vi "GetDeviceByType.vi"(8 "error in (no error)":errorcluster, 11 "DevType":i32) -> (0 "error out":errorcluster, 2 "UniqueIDs":string[](array[string]), 3 "Names":string[](array[string]))   [LabVIEW 2009]
doc: "JYGetMonos.vi\nInput - Input Error Cluster\n----------------------------------\n\nOutputs -\nUniquedIDs - string array\nDisplayNames - string array\nOutput Error Cluster\n\nUses the JYConfiguration Browser return a list\nof registered monos.\n\nThe UniqueID will be required to initialize\nthe mono"
panel:
  in  "Config Browser":refnum<k7>
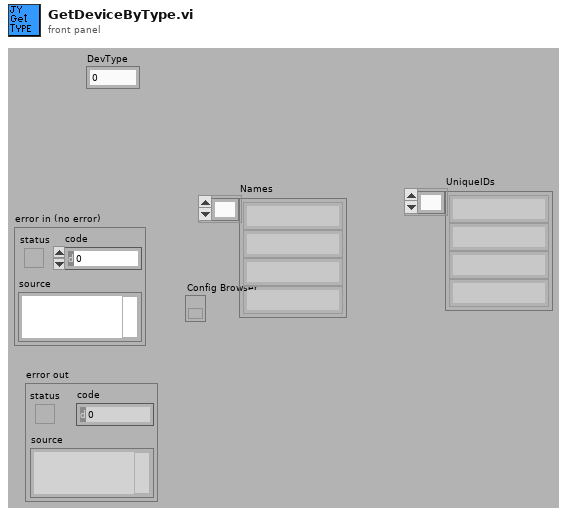
[diagram p1: front panel]
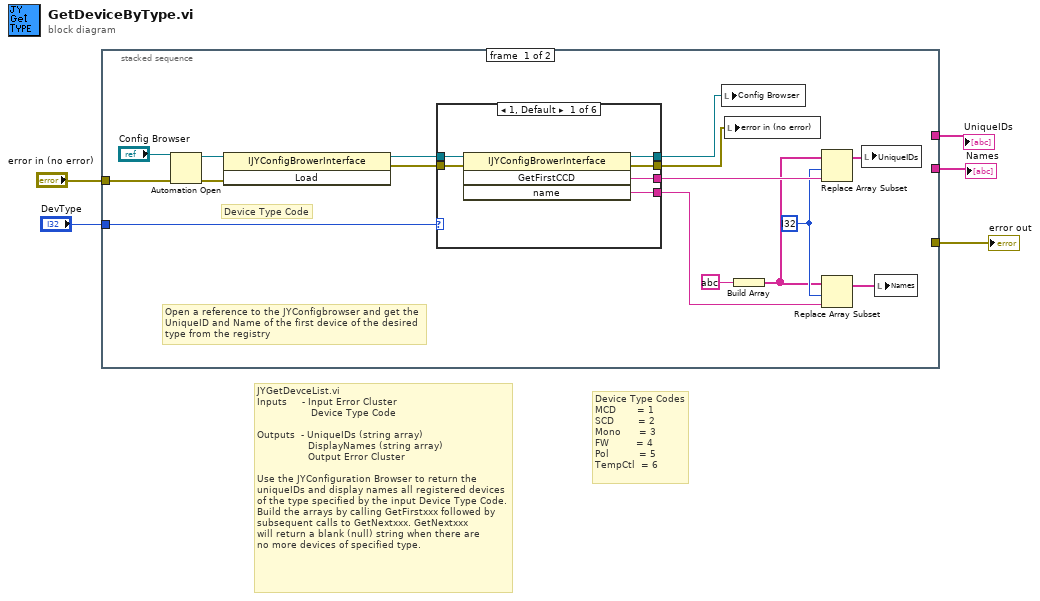
[diagram p0: block diagram]
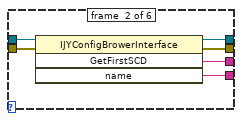
[diagram p2: hidden frame]
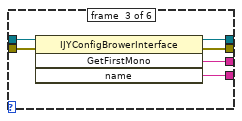
[diagram p3: hidden frame]
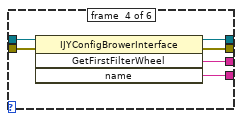
[diagram p4: hidden frame]
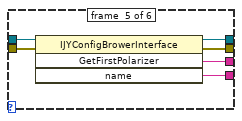
[diagram p5: hidden frame]
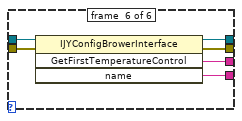
[diagram p6: hidden frame]
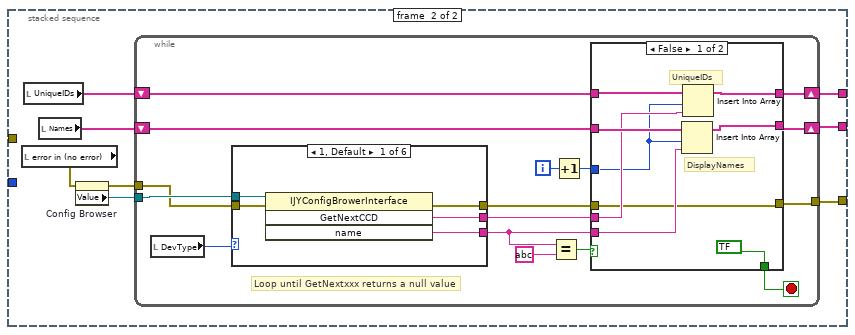
[diagram p7: hidden frame]
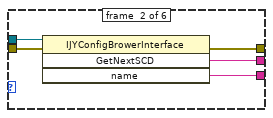
[diagram p8: hidden frame]
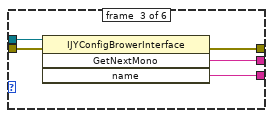
[diagram p9: hidden frame]
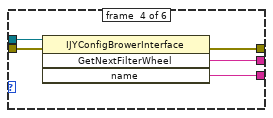
[diagram p10: hidden frame]
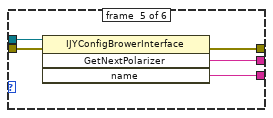
[diagram p11: hidden frame]
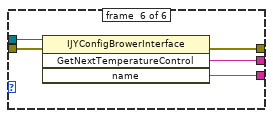
[diagram p12: hidden frame]
diagram:
  # "Device Type Codes\nMCD       = 1\nSCD        = 2\nMono      = 3\nFW         = 4\nPol          = 5\nTempCtl  = 6"
  # "JYGetDevceList.vi\nInputs     - Input Error Cluster\n                  Device Type Code\n\nOutputs  - UniqueIDs (string array)\n                 DisplayNames (string array)\n                 Output Error Cluster\n\nUse the JYConfiguration Browser to return the\nuniqueIDs and display names all registered devices\nof the type specified by the input Device Type Code.\nBuild the arrays by calling GetFirstxxx followed by\nsubsequent calls to GetNextxxx. GetNextxxx\nwill return a blank (null) string when there are\nno more devices of specified type."
  n1 = stacked-sequence {
    tunnel: [_ w60] -> w4
    tunnel: [_ w59] -> w5
    tunnel: [_ w58] -> w2
    tunnel: "error in (no error)" -> [w7 _]
    tunnel: "DevType" -> [w6 _]
    frame #0 {
      w12 = i32 ?
      # "Device Type Code"
      # "Open a reference to the JYConfigbrowser and get the\nUniqueID and Name of the first device of the desired\ntype from the registry"
      n2 = Automation Open(error in (no error)=w7, Automation Refnum="Config Browser") -> (Automation Refnum=w21:refnum<k7>, error out=w19:errorcluster)  [unwired: 2 out]
      n3 = invoke class="IJYConfigBrowerInterface" method="Load"(reference=w21, error in=w19) -> (reference out=w20:refnum<k7>, error out=w18:errorcluster)  [unwired: 1 in, 1 out]
      n4 = case shown="1, Default" w6 {
        tunnel: w20 -> [w22 w33 w39 w45 w51 w57]
        tunnel: w18 -> [w27 w32 w38 w44 w50 w56]
        tunnel: [w26 w31 w37 w43 w49 w55] -> w16
        tunnel: [w25 w30 w36 w42 w48 w54] -> w14
        tunnel: [w24 w29 w35 w41 w47 w53] -> w13
        tunnel: [w23 w28 w34 w40 w46 w52] -> w10
        frame #0 {
          n5 = invoke class="IJYConfigBrowerInterface" method="GetFirstCCD"(reference=w22, error in=w27) -> (reference out=w26:refnum<k7>, error out=w25:errorcluster, "GetFirstCCD"=w24:string, "name"=w23:string)  [unwired: 2 in]
        }
        frame #1 {
          n6 = invoke class="IJYConfigBrowerInterface" method="GetFirstSCD"(reference=w33, error in=w32) -> (reference out=w31:refnum<k7>, error out=w30:errorcluster, "GetFirstSCD"=w29:string, "name"=w28:string)  [unwired: 2 in]
        }
        frame #2 {
          n7 = invoke class="IJYConfigBrowerInterface" method="GetFirstMono"(reference=w39, error in=w38) -> (reference out=w37:refnum<k7>, error out=w36:errorcluster, "GetFirstMono"=w35:string, "name"=w34:string)  [unwired: 2 in]
        }
        frame #3 {
          n8 = invoke class="IJYConfigBrowerInterface" method="GetFirstFilterWheel"(reference=w45, error in=w44) -> (reference out=w43:refnum<k7>, error out=w42:errorcluster, "GetFirstFilterWheel"=w41:string, "name"=w40:string)  [unwired: 2 in]
        }
        frame #4 {
          n9 = invoke class="IJYConfigBrowerInterface" method="GetFirstPolarizer"(reference=w51, error in=w50) -> (reference out=w49:refnum<k7>, error out=w48:errorcluster, "GetFirstPolarizer"=w47:string, "name"=w46:string)  [unwired: 2 in]
        }
        frame #5 {
          n10 = invoke class="IJYConfigBrowerInterface" method="GetFirstTemperatureControl"(reference=w57, error in=w56) -> (reference out=w55:refnum<k7>, error out=w54:errorcluster, "GetFirstTemperatureControl"=w53:string, "name"=w52:string)  [unwired: 2 in]
        }
      }
      n11 = local write "Config Browser"(w16) -> ()
      n12 = local write "error in (no error)"(w14) -> ()
      n13 = Build Array(string ?) -> (w11:string[])
      n14 = Replace Array Subset(array=w11, new element=w13, index=w12) -> (w9:string[])
      n15 = Replace Array Subset(array=w11, new element=w10, index=w12) -> (w8:string[])
      n16 = local write "UniqueIDs"(w9) -> ()
      n17 = local write "Names"(w8) -> ()
    }
    frame #1 {
      n18 = local read "error in (no error)"() -> (w64:errorcluster)
      n19 = local read "UniqueIDs"() -> (w62:string[])
      n20 = local read "Names"() -> (w61:string[])
      n21 = property on="Config Browser" class="Ref (strict)"(error in=w64) -> (error out=w63:errorcluster, "Value"=w65:refnum<k7>)  [unwired: 1 in, 1 out]
      n22 = while {
        tunnel: w65 -> [w81]
        tunnel: w63 -> [w80]
        shift-right: [w67] -> w60
        shift-left: w62 -> [w68]
        shift-right: [w74] -> w59
        shift-left: w61 -> [w75]
        tunnel: [w69] -> w58
        i -> [w79]
        stop <- w76 stop-if-true
        # "Loop until GetNextxxx returns a null value"
        n23 = local read "DevType"() -> (w66:i32)
        n24 = case shown="1, Default" w66 {
          tunnel: w81 -> [w86 w91 w96 w101 w106 w111]
          tunnel: w80 -> [w85 w90 w95 w100 w105 w110]
          tunnel: [w84 w89 w94 w99 w104 w109] -> w73
          tunnel: [w83 w88 w93 w98 w103 w108] -> w72
          tunnel: [w82 w87 w92 w97 w102 w107] -> w70
          frame #0 {
            n25 = invoke class="IJYConfigBrowerInterface" method="GetNextCCD"(reference=w86, error in=w85) -> (error out=w82:errorcluster, "GetNextCCD"=w84:string, "name"=w83:string)  [unwired: 2 in, 1 out]
          }
          frame #1 {
            n26 = invoke class="IJYConfigBrowerInterface" method="GetNextSCD"(reference=w91, error in=w90) -> (error out=w87:errorcluster, "GetNextSCD"=w89:string, "name"=w88:string)  [unwired: 2 in, 1 out]
          }
          frame #2 {
            n27 = invoke class="IJYConfigBrowerInterface" method="GetNextMono"(reference=w96, error in=w95) -> (error out=w92:errorcluster, "GetNextMono"=w94:string, "name"=w93:string)  [unwired: 2 in, 1 out]
          }
          frame #3 {
            n28 = invoke class="IJYConfigBrowerInterface" method="GetNextFilterWheel"(reference=w101, error in=w100) -> (error out=w97:errorcluster, "GetNextFilterWheel"=w99:string, "name"=w98:string)  [unwired: 2 in, 1 out]
          }
          frame #4 {
            n29 = invoke class="IJYConfigBrowerInterface" method="GetNextPolarizer"(reference=w106, error in=w105) -> (error out=w102:errorcluster, "GetNextPolarizer"=w104:string, "name"=w103:string)  [unwired: 2 in, 1 out]
          }
          frame #5 {
            n30 = invoke class="IJYConfigBrowerInterface" method="GetNextTemperatureControl"(reference=w111, error in=w110) -> (error out=w107:errorcluster, "GetNextTemperatureControl"=w109:string, "name"=w108:string)  [unwired: 2 in, 1 out]
          }
        }
        n31 = Equal?(x=w72, y=string ?) -> (x = y?=w77:bool)
        n32 = Increment(x=w79) -> (x+1=w71:i32)
        n33 = case shown="False" w77 {
          selector: w77 -> [_ w124]
          tunnel: [bool ? w124] -> w76
          tunnel: w68 -> [w113 w122]
          tunnel: w75 -> [w119 w121]
          tunnel: [w115 w121] -> w74
          tunnel: w73 -> [w118 _]
          tunnel: w72 -> [w117 _]
          tunnel: w71 -> [w116 _]
          tunnel: w70 -> [w114 w123]
          tunnel: [w114 w123] -> w69
          tunnel: [w112 w122] -> w67
          frame #0 {
            # "DisplayNames"
            # "UniqueIDs"
            n34 = Insert Into Array(array=w119, index=w116, new element=w117) -> (w115:string[])
            n35 = Insert Into Array(array=w113, index=w116, new element=w118) -> (w112:string[])
          }
          frame #1 {
            # "Null value returned -\nno more monos - quit"
          }
        }
      }
    }
  }
  "UniqueIDs" <- w4
  "Names" <- w5
  "error out" <- w2
